vi "calculate fly.vi"(8 "error in (no error)":errorcluster, 10 "distance":dbl, 11 "direction":u16) -> (0 "error out":errorcluster)   [LabVIEW 2015, in "SCANalone4x64.lvlib"]
doc: "__declspec(dllimport) void __stdcall calculate_fly(unsigned short direction, double distance);"
uses:
  <userlib>/SCANalone4x64/SCANalone4x64.lvlib
  <userlib>/SCANalone4x64/SCANalone4x64.dll
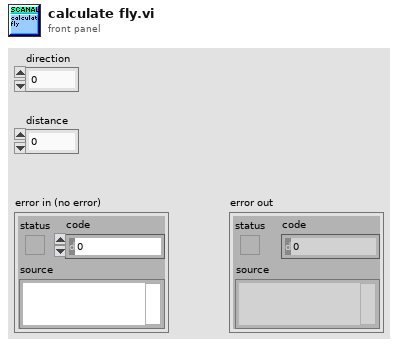
[diagram p1: front panel]
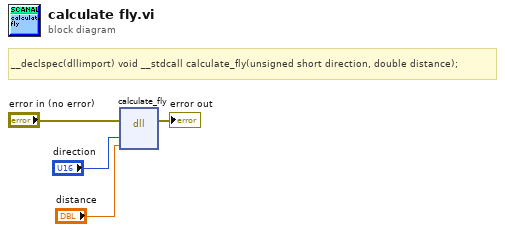
[diagram p0: block diagram]
diagram:
  # "__declspec(dllimport) void __stdcall calculate_fly(unsigned short direction, double distance);"
  n1 = dll-call lib="C:/Program Files/National Instruments/LabVIEW 2015/user.lib/SCANalone4x64/SCANalone4x64.*" fn="calculate_fly"(error in="error in (no error)", "direction"="direction", "distance"="distance") -> (error out=→"error out":errorcluster)  [unwired: 5 in, 1 out]
